vi "Latihan 19 (Isi Air Tank).vi"() -> ()   [LabVIEW 2021]
panel:
  in  "Empty":bool
  out "Tank":dbl(slide) scale=0.0..100.0
  out "empty":bool
  out "full":bool
  in  "Fill":bool
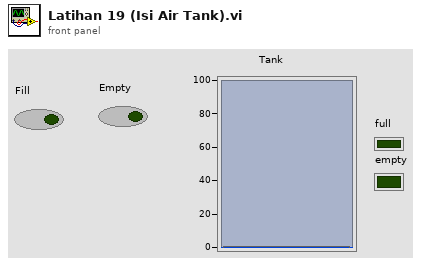
[diagram p1: front panel]
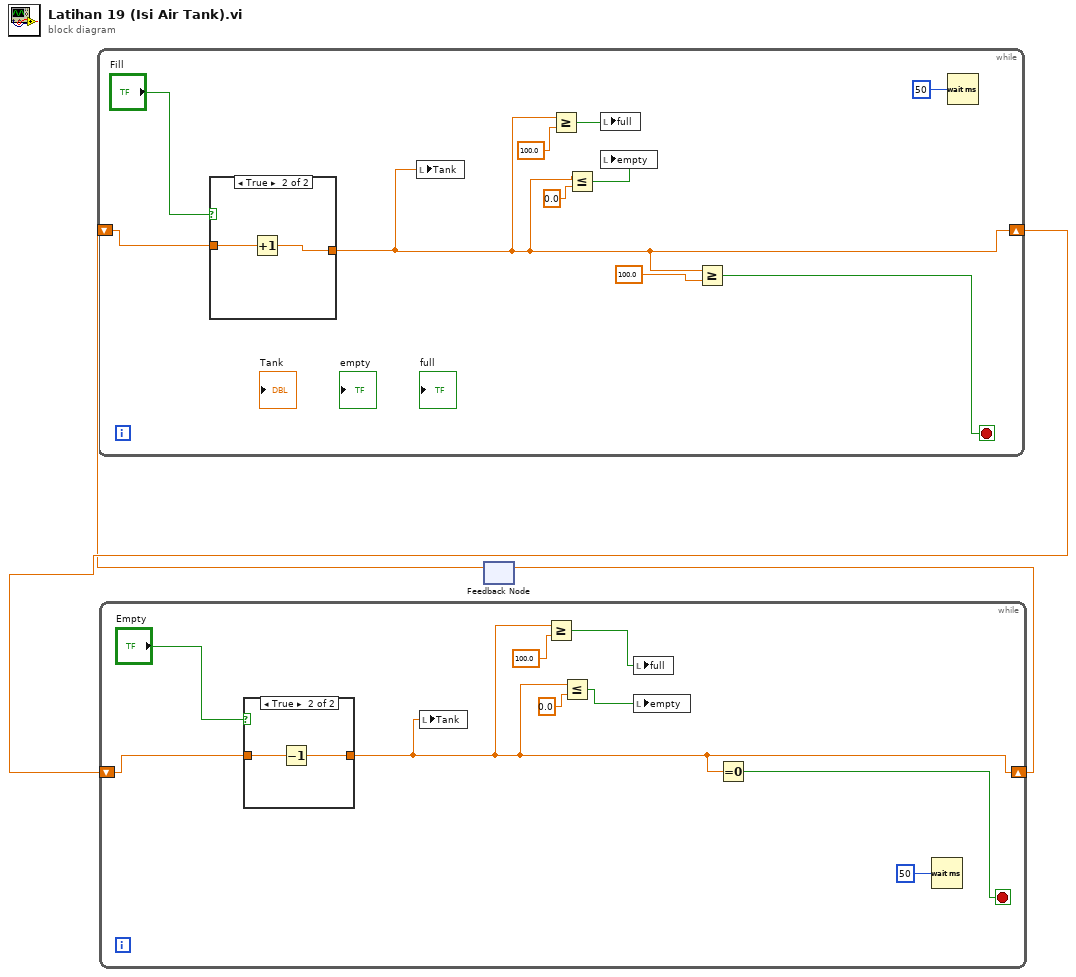
[diagram p0: block diagram]
diagram:
  n1 = feedback #1() -> (w1:dbl)  [unwired: 1 in]
  n2 = while {
    shift-right: [w7] -> w3
    shift-left: w1 -> [w13]
    stop <- w8 stop-if-true
    n3 = case shown="True" "Fill" {
      tunnel: w13 -> [w14 w16]
      tunnel: [w14 w15] -> w7
      frame False {
      }
      frame True {
        n4 = Increment(x=w16) -> (x+1=w15:dbl)
      }
    }
    n5 = local write "Tank"(w7) -> ()
    n6 = Greater Or Equal?(x=w7, y=100.0) -> (x >= y?=w10:bool)
    n7 = Less Or Equal?(x=w7, y=0.0) -> (x <= y?=w12:bool)
    n8 = local write "full"(w10) -> ()
    n9 = local write "empty"(w12) -> ()
    n10 = Greater Or Equal?(x=w7, y=100.0) -> (x >= y?=w8:bool)
    n11 = Wait (ms)(milliseconds to wait=u32 50) -> ()  [unwired: 1 out]
  }
  n12 = while {
    shift-right: [w20] -> w2
    shift-left: w3 -> [w25]
    stop <- w19 stop-if-true
    n13 = case shown="True" "Empty" {
      tunnel: w25 -> [w26 w28]
      tunnel: [w26 w27] -> w20
      frame False {
      }
      frame True {
        n14 = Decrement(x=w28) -> (x-1=w27:dbl)
      }
    }
    n15 = local write "Tank"(w20) -> ()
    n16 = Greater Or Equal?(x=w20, y=100.0) -> (x >= y?=w22:bool)
    n17 = Less Or Equal?(x=w20, y=0.0) -> (x <= y?=w21:bool)
    n18 = local write "full"(w22) -> ()
    n19 = local write "empty"(w21) -> ()
    n20 = Equal To 0?(x=w20) -> (x = 0?=w19:bool)
    n21 = Wait (ms)(milliseconds to wait=u32 50) -> ()  [unwired: 1 out]
  }
  n22 = feedback-in #1(w2) -> ()
